vi "Locate Breakdown.vi"(0 "Signals":waveform(dbl)[](array[waveform]), 7 "Offset (µs)":dbl format="%#_13g", 9 "Duration (µs)":dbl format="%#_13g", 11 "error in (no error)":errorcluster, 13 "Microphone Coordinates (cm, rad, cm)":cluster{"r":dbl, "theta":dbl, "z":dbl}[](array[cluster])) -> (4 "Coordinates (cm, rad, cm)":cluster{"r":sgl, "theta":sgl, "z":sgl}[](array[cluster]), 8 "Upstream/Downstream Delay (s)":dbl, 15 "error out":errorcluster)   [LabVIEW 2013, in "Breakdown Acoustics Controls.lvlib"]
uses:
  <vilib>/Analysis/2dsp.llb/1D Cross Correlation (DBL).vi
  <vilib>/Waveform/WDTOps.llb/WDT Get Waveform Subset DBL.vi
  <vilib>/Waveform/WDTOps.llb/WDT Index Channel DBL.vi
  Breakdown Acoustics Controls.lvlib
  <vilib>/Analysis/NI_AALPro.lvlib
panel:
  out "Sampling Rate":u16
  out "Array":i32[](array[numeric])
  out "Source Signals Correlation":dbl[](graph)
  out "Shifted Source Signals":dbl[][](graph)
  out "Downstream Signals":waveform(dbl)[](graph)
  out "Upstream Signals":waveform(dbl)[](graph)
  out "Duration (S)":dbl
  out "Offset (S)":dbl
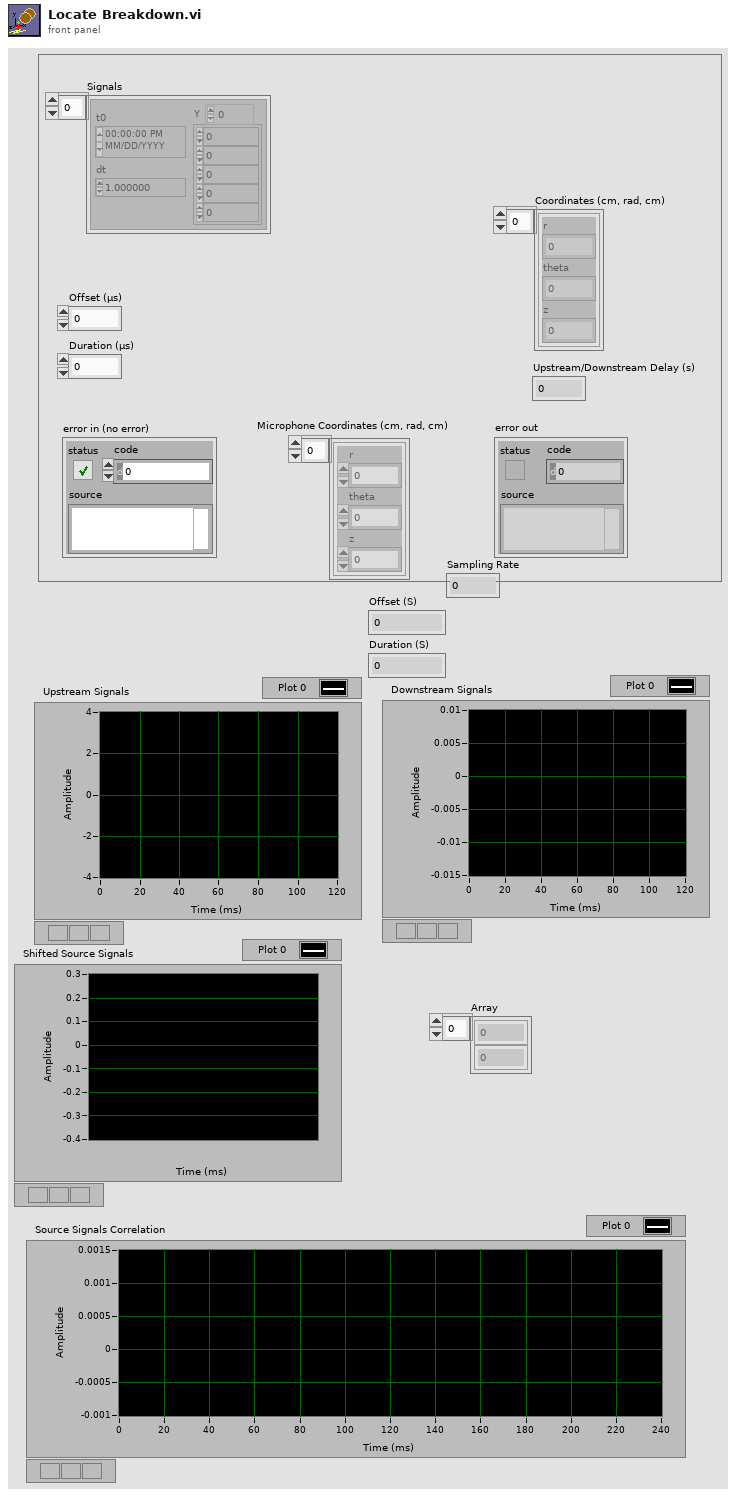
[diagram p1: front panel]
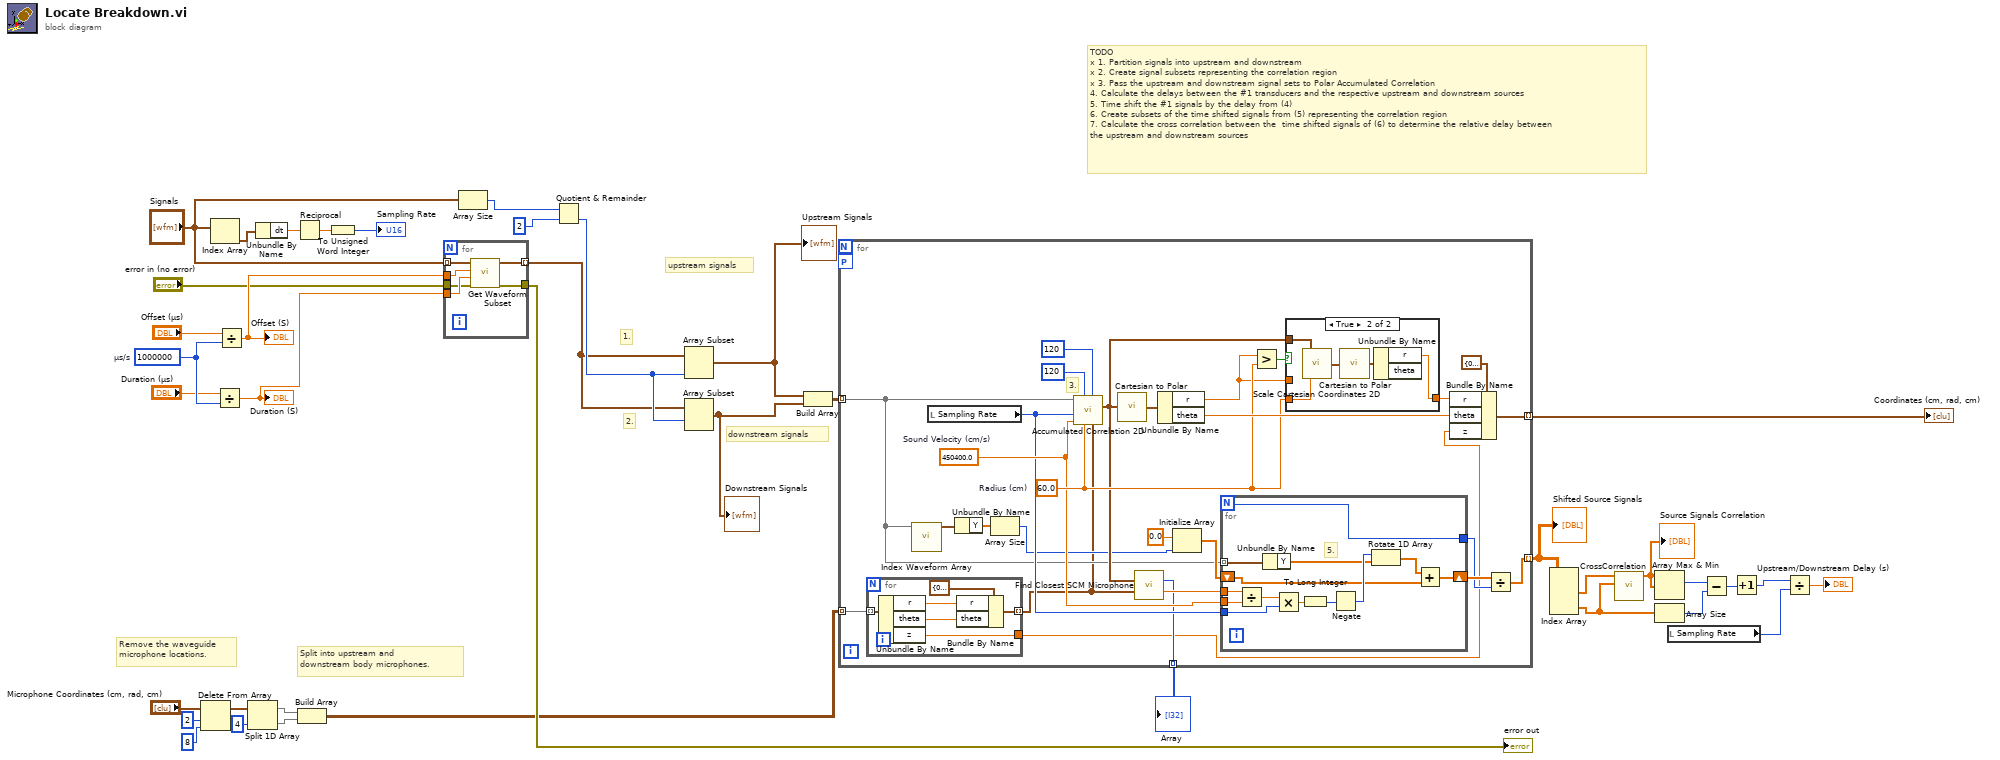
[diagram p0: block diagram]
diagram:
  w15 = 1000000  # µs/s
  # "Split into upstream and\ndownstream body microphones."
  # "Remove the waveguide\nmicrophone locations."
  # "2."
  # "1."
  # "downstream signals"
  # "upstream signals"
  # "TODO\nx 1. Partition signals into upstream and downstream\nx 2. Create signal subsets representing the correlation region\nx 3. Pass the upstream and downstream signal sets to Polar Accumulated Correlation\n4. Calculate the delays between the #1 transducers and the respective upstream and downstream sources\n5. Time shift the #1 signals by the delay from (4)\n6. Create subsets of the time shifted signals from (5) representing the correlation region\n7. Calculate the cross correlation between the  time shifted signals of (6) to determine the relative delay between\nthe upstream and downstream sources"
  n1 = Delete From Array(array="Microphone Coordinates (cm, rad, cm)", length=2, index=8) -> (array with subset deleted=w5:cluster{"r":dbl, "theta":dbl, "z":dbl}[])  [unwired: 1 out]
  n2 = Index Array(array="Signals") -> (element=w17:waveform(dbl))  [unwired: 1 in]
  n3 = Divide(x="Duration (µs)", y=w15) -> (x/y=w21:dbl)
  "Duration (S)" <- w21
  n4 = Divide(x="Offset (µs)", y=w15) -> (x/y=w22:dbl)
  "Offset (S)" <- w22
  n5 = Split 1D Array(array=w5, index=4) -> (first subarray=w3:cluster{"r":dbl, "theta":dbl, "z":dbl}[], second subarray=w2:cluster{"r":dbl, "theta":dbl, "z":dbl}[])
  n6 = Unbundle By Name(w17) -> ("dt"=w16:dbl)
  n7 = Reciprocal(x=w16) -> (1/x=w10:dbl)
  n8 = Build Array(w3, w2) -> (w1:cluster{"r":dbl, "theta":dbl, "z":dbl}[][])
  n9 = To Unsigned Word Integer(number=w10) -> (unsigned 16bit integer=→"Sampling Rate":u16)
  n10 = for {
    tunnel: "Signals" -> [w45] mode=indexing
    tunnel: [w44] -> w23 mode=indexing
    tunnel: w22 -> [w43]
    tunnel: w21 -> [w42]
    tunnel: "error in (no error)" -> [w41]
    tunnel: [w40] -> w11
    n11 = call-poly <vilib>:"Get Waveform Subset.vi"("error in (no error)"=w41, "duration"=w42, "start samples/time"=w43, "waveform in"=w45) -> ("error out"=w40:errorcluster, "waveform out"=w44:waveform(dbl))  [unwired: 2 in, 2 out]
  }
  "error out" <- w11
  n12 = Array Size(array="Signals") -> (size(s)=w19:i32)
  n13 = Quotient & Remainder(x=w19, y=2) -> (floor(x/y)=w30:i32)  [unwired: 1 out]
  n14 = Array Subset(array=w23, length=w30) -> (w20:waveform(dbl)[])  [unwired: 1 in]
  "Upstream Signals" <- w20
  n15 = Array Subset(array=w23, index=w30) -> (w29:waveform(dbl)[])  [unwired: 1 in]
  "Downstream Signals" <- w29
  n16 = Build Array(w20, w29) -> (w39:waveform(dbl)[][])
  n17 = for {
    tunnel: w39 -> [w50] mode=indexing
    tunnel: w1 -> [w48] mode=indexing
    tunnel: [w70] -> w32 mode=indexing
    tunnel: [w57] -> w26 mode=indexing
    workers-P: _ -> [_]
    tunnel: [w58] -> w24 mode=indexing
    w64 = 60.0  # Radius (cm)
    w60 = 450400.0  # Sound Velocity (cm/s)
    # "3."
    n18 = for {
      tunnel: w48 -> [w78] mode=indexing
      tunnel: [w77] -> w46
      tunnel: [w73] -> w47 mode=indexing
      n19 = Unbundle By Name(w78) -> ("r"=w75:dbl, "theta"=w74:dbl, "z"=w77:dbl)
      n20 = Bundle By Name(cluster=cluster{"r":dbl, "theta":dbl} {"r"=0.0, "theta"=0.0} ("Polar\nCoordinates"), "r"=w75, "theta"=w74) -> (w73:cluster{"r":dbl, "theta":dbl})
    }
    n21 = call-poly <vilib>:"Index Waveform Array.vi"("waveform array"=w50) -> ("waveform"=w52:waveform(dbl))  [unwired: 9 in, 1 out]
    n22 = local read "Sampling Rate"() -> (w59:u16)
    n23 = Unbundle By Name(w52) -> ("Y"=w51:dbl[])
    n24 = Array Size(array=w51) -> (size(s)=w49:i32)
    n25 = call "Accumulated Correlation 2D.vi"("Microphone Coordinates (cm, rad)"=w47, "Ny"=120 ("Ntheta"), "Radius (cm)"=w64, "Nx"=120 ("Nr"), "Sound Velocity (cm/s)"=w60, "Sampling Rate"=w59, "Waveforms"=w50) -> ("Source Coordinates (cm, cm)"=w62:cluster{"x":dbl, "y":dbl})  [unwired: 4 in]
    n26 = call "Cartesian to Polar.vi"("Cartesian\nCoordinates"=w62) -> ("Polar\nCoordinates"=w69:cluster{"r":dbl, "theta":dbl})  [unwired: 4 in]
    n27 = call "Find Closest SCM Microphone.vi"("Source Polar\nCoordinates"=w62, "Microphone Coordinates (cm, rad)"=w47) -> ("Closest Microphone Index"=w58:i32, "Closest Microphone Distance (cm)"=w61:dbl)  [unwired: 12 in]
    n28 = Unbundle By Name(w69) -> ("r"=w63:dbl, "theta"=w68:dbl)
    n29 = Initialize Array(0.0 ("element"), w49) -> (w53:dbl[])
    n30 = for {
      N -> [w82]
      tunnel: w61 -> [w91]
      tunnel: w60 -> [w90]
      tunnel: w59 -> [w88]
      tunnel: w50 -> [w80] mode=indexing
      shift-right: [w83] -> w56
      shift-left: w53 -> [w81]
      tunnel: [w82] -> w55
      # "5."
      n31 = Divide(x=w91, y=w90) -> (x/y=w89:dbl)
      n32 = Unbundle By Name(w80) -> ("Y"=w79:dbl[])
      n33 = Multiply(x=w89, y=w88) -> (x*y=w87:dbl)
      n34 = To Long Integer(number=w87) -> (32bit integer=w86:i32)
      n35 = Negate(x=w86) -> (-x=w85:i32)
      n36 = Rotate 1D Array(1:w79, 2:w85) -> (0:w84:dbl[])
      n37 = Add(x=w84, y=w81) -> (x+y=w83:dbl[])
    }
    n38 = Greater?(x=w63, y=w64) -> (0:w66:bool)
    n39 = case shown="True" w66 {
      tunnel: w64 -> [_ w96]
      tunnel: [w92 w93] -> w65
      tunnel: w62 -> [_ w97]
      tunnel: w63 -> [w92 _]
      frame False {
      }
      frame True {
        n40 = call "Scale Cartesian Coordinates 2D.vi"("Max Radius"=w96, "Source Coordinates (cm, cm)"=w97) -> ("output cluster"=w95:cluster{"x":dbl, "y":dbl})  [unwired: 3 in]
        n41 = call "Cartesian to Polar.vi"("Cartesian\nCoordinates"=w95) -> ("Polar\nCoordinates"=w94:cluster{"r":dbl, "theta":dbl})  [unwired: 4 in]
        n42 = Unbundle By Name(w94) -> ("r"=w93:dbl)  [unwired: 1 out]
      }
    }
    n43 = Bundle By Name(cluster=cluster{"r":sgl, "theta":sgl, "z":sgl} {"r"=0.0, "theta"=0.0, "z"=0.0} ("Coordinates (m)"), "r"=w65, "theta"=w68, "z"=w46) -> (w70:cluster{"r":sgl, "theta":sgl, "z":sgl})
    n44 = Divide(x=w56, y=w55) -> (x/y=w57:dbl[])
  }
  "Coordinates (cm, rad, cm)" <- w32
  "Shifted Source Signals" <- w26
  "Array" <- w24
  n45 = Index Array(array=w26) -> (element #1=w28:dbl[], element #2=w27:dbl[])  [unwired: 4 in]
  n46 = call-poly <vilib>:"CrossCorrelation.vi"("Y"=w27, "X"=w28) -> ("Rxy"=w25:dbl[])  [unwired: 8 in, 1 out]
  "Source Signals Correlation" <- w25
  n47 = Array Max & Min(array=w25) -> (max index (indices)=w38:i32)  [unwired: 3 out]
  n48 = Array Size ("Size(s)")(array=w27) -> (size(s)=w37:i32)
  n49 = local read "Sampling Rate"() -> (w34:u16)
  n50 = Subtract(x=w38, y=w37) -> (x-y=w36:i32)
  n51 = Increment(x=w36) -> (x+1=w35:i32)
  n52 = Divide(x=w35, y=w34) -> (x/y=→"Upstream/Downstream Delay (s)":dbl)
